vi "Make servo signal.vi"(4 "midpoint (ms)":dbl=1.5, 5 "A":dbl=1.2727, 6 "scale (ms/deg)":dbl=0.01666666666667, 7 "b":dbl=-0.169, 10 "sampling frequency":dbl=50.0, 11 "Data":dbl[](array[numeric])) -> (1 "compensated":dbl[](array[numeric]), 2 "out of range":bool, 3 "sine PWM pattern":cluster{"duty cycle":dbl, "frequency":dbl}[](array[cluster]))   [LabVIEW 2013]
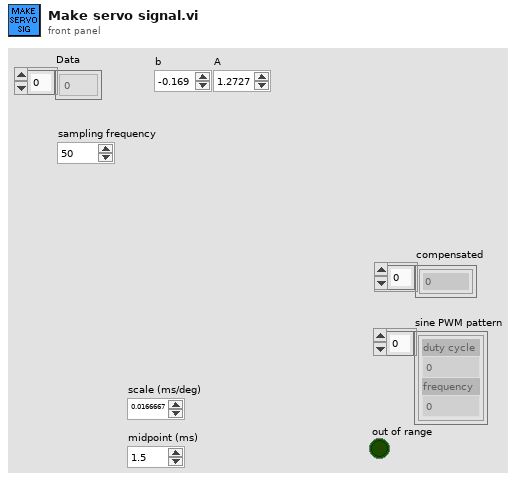
[diagram p1: front panel]
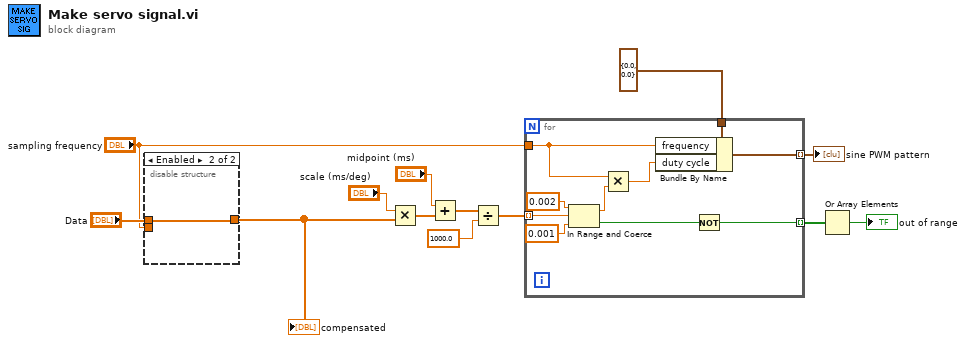
[diagram p0: block diagram]
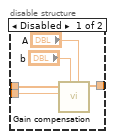
[diagram p2: hidden frame]
diagram:
  n1 = disable-structure shown="Enabled" {
    disable-tunnel: "Data" -> [w18 w19]
    disable-tunnel: [w17 w19] -> w3
    disable-tunnel: "sampling frequency" -> [w16 _]
    frame Disabled {
      n2 = call "Gain compensation.vi"("A"="A", "b"="b", "sampling frequency"=w16, "Data"=w18) -> ("compensated"=w17:dbl[])  [unwired: 7 in]
    }
    frame Enabled {
    }
  }
  "compensated" <- w3
  n3 = Multiply(x="scale (ms/deg)", y=w3) -> (x*y=w12:dbl[])
  n4 = Add(x="midpoint (ms)", y=w12) -> (x+y=w7:dbl[])
  n5 = Divide(x=w7, y=1000.0 ("cycles")) -> (x/y=w6:dbl[])
  n6 = for {
    tunnel: w6 -> [w26] mode=indexing
    tunnel: "sampling frequency" -> [w29]
    tunnel: [w27] -> w1 mode=indexing
    tunnel: [w21] -> w9 mode=indexing
    tunnel: cluster{"duty cycle":dbl, "frequency":dbl} {"duty cycle"=0.0, "frequency"=0.0} ("values") -> [w20]
    n7 = In Range and Coerce(upper limit=0.002, x=w26, lower limit=0.001) -> (coerced(x)=w23:dbl, In Range?=w22:bool)
    n8 = Multiply(x=w29, y=w23) -> (x*y=w28:dbl)
    n9 = Bundle By Name(cluster=w20, "frequency"=w29, "duty cycle"=w28) -> (w27:cluster{"duty cycle":dbl, "frequency":dbl})
    n10 = Not(x=w22) -> (.not. x?=w21:bool)
  }
  "sine PWM pattern" <- w1
  n11 = Or Array Elements(Boolean array=w9) -> (logical OR=→"out of range":bool)
